vi "test.vi"() -> ()   [LabVIEW 2016]
panel:
  out "层数 2":string
  out "层数参数位置 2":i32
  out "总包数 2":i32
  out "当前包号 2":i32
  out "小时数据发送次数":i32
  out "大小":i32
  out "总包数":i32[](array[numeric])
  out "当前包号":i32[](array[numeric])
  out "行数":i32[](array[numeric])
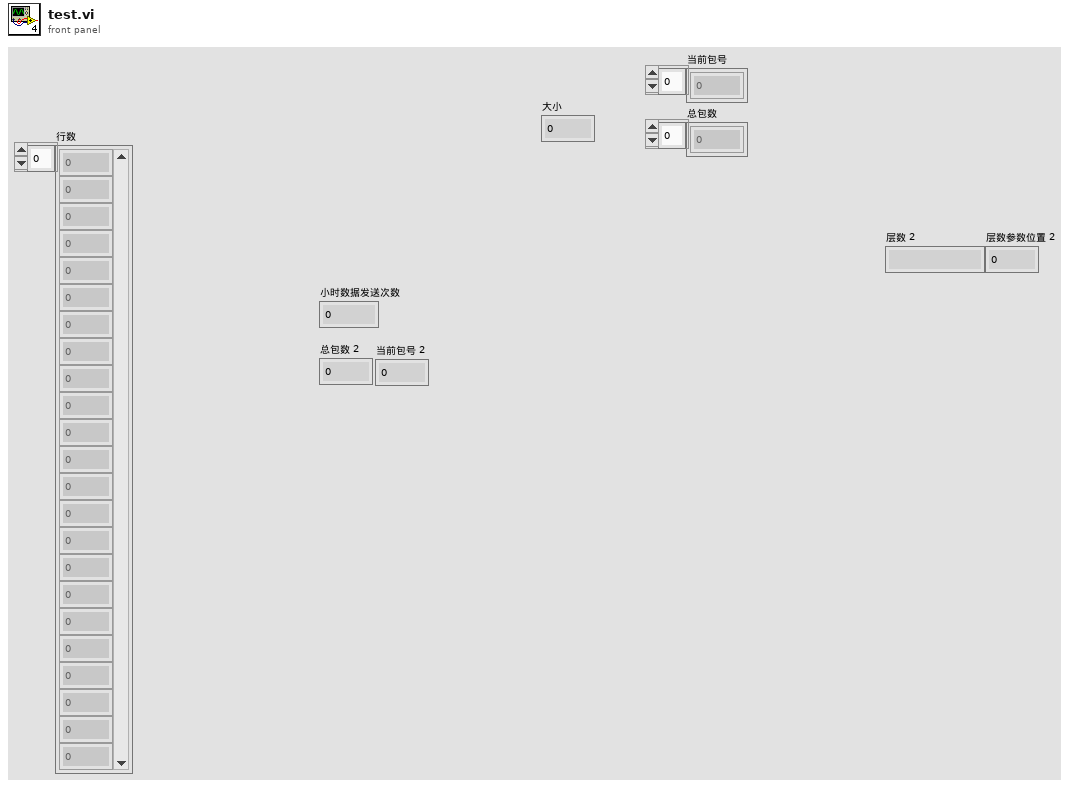
[diagram p1: front panel]
types:
  T1 = cluster{"CODMn":string, "CODCr":string, "DO":string, "铜":string, "PH":string, "氨氮":string, "比电导率":string, "水温":string, "COD":string, "浊度":string, "总氮":string, "总磷":string, "叶绿素a":string, "藻密度":string, "水位":string, "流速":string, "方向":string, "瞬时流量":string, "累积流量":string, "正累积流量":string, "负累积流量":string, "亚硝酸盐":string, "硫化物":string, "ORP":string, "铅":string, "镉":string, "锌":string, "镍":string, "锰":string, "汞":string, "气温":string, "气压":string, "风速":string, "风向":string, "空气温度":string, "相对湿度":string, "分钟雨量":string, "小时雨量":string, "日雨量":string, "累积雨量":string, "盐度":string, "磷酸盐":string, "硝氮":string, "氟化物":string, "挥发酚":string, "氯化物":string, "蓝绿藻":string, "余氯":string, "综合生物毒性":string, "艏向":string, "横摇":string, "纵摇":string, "分层标志":string, "层状态1":string, "层状态2":string, "水平平均流速":string, "流向":string, "北向流速分量":string, "东向流速分量":string, "垂直流速分量":string, "最大波高":string, "最大波周期":string, "1/10波高":string, "1/10波周期":string, "有效波高":string, "有效波周期":string, "平均波高":string, "平均波周期":string, "波向":string, "波个数":string, "水深":string}
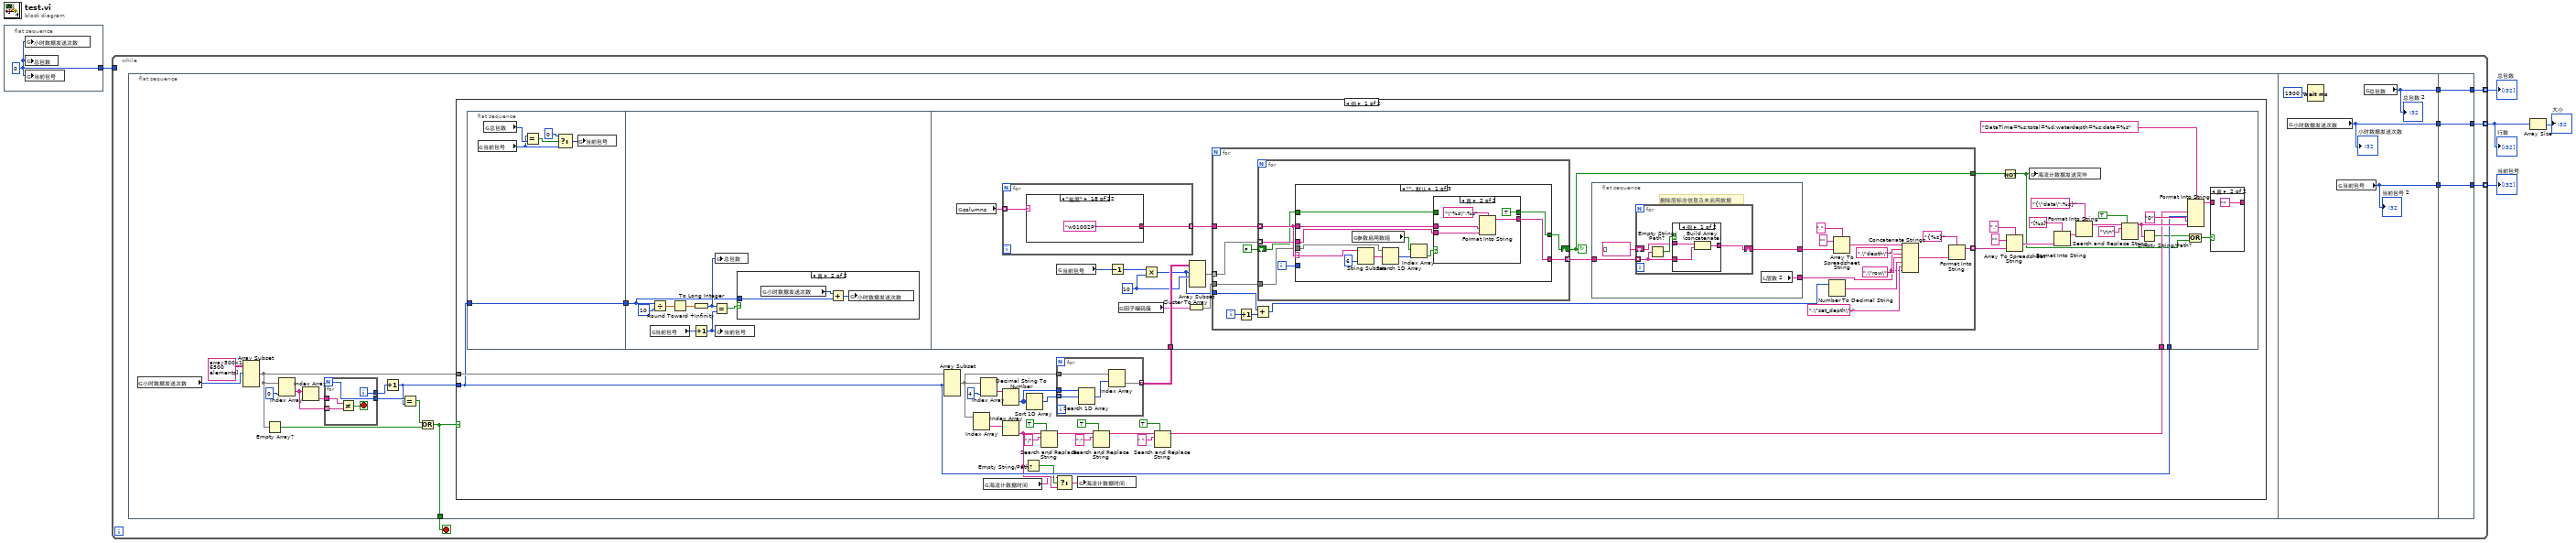
[diagram p0: block diagram]
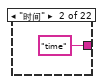
[diagram p5: hidden frame]
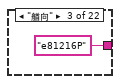
[diagram p6: hidden frame]
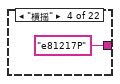
[diagram p7: hidden frame]
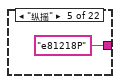
[diagram p8: hidden frame]
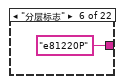
[diagram p9: hidden frame]
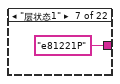
[diagram p10: hidden frame]
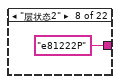
[diagram p11: hidden frame]
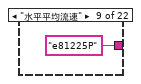
[diagram p12: hidden frame]
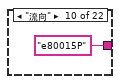
[diagram p13: hidden frame]
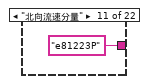
[diagram p14: hidden frame]
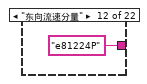
[diagram p15: hidden frame]
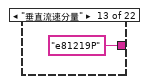
[diagram p16: hidden frame]
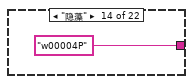
[diagram p17: hidden frame]
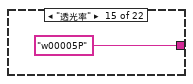
[diagram p18: hidden frame]
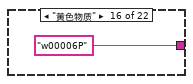
[diagram p19: hidden frame]
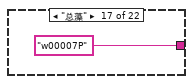
[diagram p20: hidden frame]
diagram:
  n1 = flat-sequence {
    tunnel: [w6] -> w1
    frame #0 {
      w6 = 0 ("小时数据发送次数")
      n2 = global write "全局 小时数据发送次数.vi" "小时数据发送次数"(w6) -> ()
      n3 = global write "全局 数据数组大小.vi" "总包数"(w6) -> ()
      n4 = global write "全局 数据数组大小.vi" "当前包号"(w6) -> ()
    }
  }
  n5 = while {
    tunnel: [w12] -> w3 mode=indexing
    tunnel: [w11] -> w5 mode=indexing
    tunnel: [w10] -> w4 mode=indexing
    tunnel: w1 -> [_]
    stop <- w13 stop-if-true
    n6 = flat-sequence {
      tunnel: [w14] -> w13
      tunnel: [w209] -> w9
      tunnel: [w208] -> w8
      tunnel: [w207] -> w7
      tunnel: [w210] -> w10
      tunnel: [w211] -> w11
      tunnel: [w212] -> w12
      tunnel: w9 -> [w212]
      tunnel: w8 -> [w211]
      tunnel: w7 -> [w210]
      frame #0 {
        n7 = global read "全局 小时数据发送次数.vi" "小时数据发送次数"() -> (w25:i32)
        n8 = Array Subset(array=string[][] array500x13[6500 elements] ("data"), index (row)=w25) -> (w15:string[][])  [unwired: 3 in]
        n9 = Empty Array?(array=w15) -> (empty?=w17:bool)
        n10 = Index Array(array=w15, index (col)=0 ("禁用的索引 (列)")) -> (element=w23:string[])  [unwired: 1 in]
        n11 = Index Array(array=w23) -> (element=w22:string)  [unwired: 1 in]
        n12 = for {
          N -> [w201]
          tunnel: w23 -> [w204] mode=indexing
          tunnel: w22 -> [w205]
          tunnel: [w202] -> w21
          tunnel: [w201] -> w20
          i -> [w202]
          stop <- w203 stop-if-true
          n13 = Not Equal?(x=w205, y=w204) -> (x != y?=w203:bool)
        }
        n14 = Increment(x=w21) -> (x+1=w19:i32)
        n15 = Equal?(x=w20, y=w19) -> (x = y?=w16:bool)
        n16 = Or(x=w16, y=w17) -> (x .or. y?=w14:bool)
        n17 = case shown="假" w14 {
          tunnel: w19 -> [w41 _]
          tunnel: w15 -> [w47 _]
          frame False {
            n18 = flat-sequence {
              tunnel: w41 -> [w54]
              tunnel: [w54] -> w48
              tunnel: w48 -> [w60]
              tunnel: w43 -> [w100]
              tunnel: w41 -> [w77]
              tunnel: w26 -> [w76]
              frame #0 {
                n19 = global read "全局 数据数组大小.vi" "当前包号"() -> (w57:i32)
                n20 = global read "全局 数据数组大小.vi" "总包数"() -> (w59:i32)
                n21 = Equal?(x=w57, y=w59) -> (x = y?=w58:bool)
                n22 = Select(t=0, s=w58, f=w57) -> (s? t:f=w55:i32)
                n23 = global write "全局 数据数组大小.vi" "当前包号"(w55) -> ()
              }
              frame #1 {
                n24 = global read "全局 数据数组大小.vi" "当前包号"() -> (w64:i32)
                n25 = Divide(x=w60, y=10) -> (x/y=w66:dbl)
                n26 = Round Toward +Infinity(x=w66) -> (ceil(x): smallest int >= x=w67:dbl)
                n27 = To Long Integer(number=w67) -> (32bit integer=w63:i32)
                n28 = Increment(x=w64) -> (x+1=w62:i32)
                n29 = Equal?(x=w63, y=w62) -> (x = y?=w61:bool)
                n30 = global write "全局 数据数组大小.vi" "总包数"(w63) -> ()
                n31 = global write "全局 数据数组大小.vi" "当前包号"(w62) -> ()
                n32 = case shown="真" w61 {
                  tunnel: w60 -> [_ w69]
                  frame False {
                  }
                  frame True {
                    n33 = global read "全局 小时数据发送次数.vi" "小时数据发送次数"() -> (w70:i32)
                    n34 = Add(x=w70, y=w69) -> (x+y=w68:i32)
                    n35 = global write "全局 小时数据发送次数.vi" "小时数据发送次数"(w68) -> ()
                  }
                }
              }
              frame #2 {
                w97 = 10 ("长度")
                n36 = global read "全局 所有参数.vi" "columns"() -> (w93:string[])
                n37 = for {
                  tunnel: w93 -> [w104] mode=indexing
                  tunnel: [w103] -> w92 mode=indexing
                  n38 = case shown="\"盐度\"" w104 {
                    tunnel: [_ "time" ("元素") "e81216P" "e81217P" "e81218P" "e81220P" "e81221P" "e81222P" "e81225P" "e80015P" "e81223P" "e81224P" "e81219P" "w00004P" "w00005P" "w00006P" "w00007P" "w01002P" "w01022P" "w81024P" "w81025P" "w81023P"] -> w103
                    frame "", Default {
                    }
                    frame "时间" {
                    }
                    frame "艏向" {
                    }
                    frame "横摇" {
                    }
                    frame "纵摇" {
                    }
                    frame "分层标志" {
                    }
                    frame "层状态1" {
                    }
                    frame "层状态2" {
                    }
                    frame "水平平均流速" {
                    }
                    frame "流向" {
                    }
                    frame "北向流速分量" {
                    }
                    frame "东向流速分量" {
                    }
                    frame "垂直流速分量" {
                    }
                    frame "隐藻" {
                    }
                    frame "透光率" {
                    }
                    frame "黄色物质" {
                    }
                    frame "总藻" {
                    }
                    frame "盐度" {
                    }
                    frame "蓝绿藻" {
                    }
                    frame "Fv/Fm" {
                    }
                    frame "PAR" {
                    }
                    frame "GPP" {
                    }
                  }
                }
                n39 = global read "全局 数据数组大小.vi" "当前包号"() -> (w99:i32)
                n40 = Decrement(x=w99) -> (x-1=w98:i32)
                n41 = global read "断电保存全局.vi" "因子编码簇"() -> (w96:T1)
                n42 = Multiply(x=w98, y=w97) -> (x*y=w91:i32)
                n43 = Cluster To Array(cluster=w96) -> (array=w95:string[])
                n44 = Array Subset(array=w100, index (row)=w91, length (row)=w97) -> (w94:string[][])  [unwired: 2 in]
                n45 = for {
                  tunnel: w94 -> [w146] mode=indexing
                  tunnel: w92 -> [w147]
                  tunnel: [w142] -> w78 mode=indexing
                  tunnel: w95 -> [w129]
                  tunnel: [w127] -> w75
                  tunnel: w91 -> [w126]
                  i -> [w141]
                  stop <- w127 continue-if-true
                  n46 = Increment(x=w141) -> (x+1=w133:i32)
                  n47 = Add(x=w126, y=w133) -> (x+y=w134:i32)
                  n48 = for {
                    tunnel: w147 -> [w165] mode=indexing
                    tunnel: w146 -> [w164] mode=indexing
                    tunnel: [w166] -> w132 mode=indexing
                    tunnel: w129 -> [w162]
                    shift-right: [w160] -> w127
                    shift-left: FALSE -> [w161]
                    i -> [w163]
                    n49 = case shown="\"\", 默认" w165 {
                      selector: w165 -> [w170 _ _]
                      tunnel: [w178 "" w199] -> w166
                      tunnel: w165 -> [w177 w190 w198]
                      tunnel: w164 -> [w176 w189 w194]
                      tunnel: w163 -> [_ w188 _]
                      tunnel: w162 -> [w175 _ _]
                      tunnel: w161 -> [w171 w186 w192]
                      tunnel: [w172 w186 w192] -> w160
                      frame "", Default {
                        n50 = global read "断电保存全局.vi" "参数启用数组"() -> (w174:bool[])
                        n51 = String Subset(string=w170, length (rest)=6 ("长度（剩余）")) -> (substring=w168:string)  [unwired: 1 in]
                        n52 = Search 1D Array(1D array=w175, element=w168) -> (index of element=w173:i32)  [unwired: 1 in]
                        n53 = Index Array(array=w174, index=w173) -> (element=w167:bool)
                        n54 = case shown="真" w167 {
                          tunnel: ["" w184] -> w178
                          tunnel: w177 -> [_ w183]
                          tunnel: w176 -> [_ w182]
                          tunnel: [w179 TRUE] -> w172
                          tunnel: w171 -> [w179 _]
                          frame False {
                          }
                          frame True {
                            n55 = Format Into String(format string="\"%s\":%s" ("格式字符串"), w183, w182) -> (resulting string=w184:string)  [unwired: 2 in, 1 out]
                          }
                        }
                      }
                      frame "e81220P" {
                        n56 = Format Into String(format string="\"%s\":%s" ("格式字符串"), w190, w189) -> ()  [unwired: 2 in, 2 out]
                        "层数 2" <- w189
                        "层数参数位置 2" <- w188
                      }
                      frame "time" {
                        n57 = Search and Replace String(replace all?=TRUE ("替换全部？(F)"), input string=w194, search string="/" ("搜索字符串"), replace string="-" ("替换字符串(\"\")")) -> (result string=w193:string)  [unwired: 4 in, 3 out]
                        n58 = Format Into String(format string="\"%s\":\"%s\"" ("格式字符串"), w198, w193) -> (resulting string=w199:string)  [unwired: 2 in, 1 out]
                      }
                    }
                  }
                  n59 = flat-sequence {
                    tunnel: w132 -> [w150]
                    tunnel: [w151] -> w131
                    tunnel: [w148] -> w130
                    frame #0 {
                      # "删除层标志信息及未启用数据"
                      n60 = for {
                        tunnel: w150 -> [w152] mode=indexing
                        shift-right: [w153] -> w148
                        shift-left: string[] [] -> [w154]
                        n61 = Empty String/Path?(string/path=w152) -> (empty?=w155:bool)
                        n62 = case shown="假" w155 {
                          tunnel: [w156 w159] -> w153
                          tunnel: w154 -> [w158 w159]
                          tunnel: w152 -> [w157 _]
                          frame False {
                            n63 = Build Array (concatenate)(w158, w157) -> (w156:string[])
                          }
                          frame True {
                          }
                        }
                      }
                      n64 = local read "层数 2"() -> (w151:string)
                    }
                  }
                  n65 = Number To Decimal String(number=w134) -> (decimal integer string=w138:string)  [unwired: 1 in]
                  n66 = Array To Spreadsheet String(delimiter (Tab)="," ("分隔符(Tab)"), array=w130, 3:"" ("格式字符串")) -> (spreadsheet string=w136:string)
                  n67 = Concatenate Strings(w136, ",\"depth\":", w131, ",\"row\":", w138, ",\"set_depth\":", w131) -> (w135:string)
                  n68 = Format Into String(format string="{%s}" ("格式字符串"), w135) -> (resulting string=w142:string)  [unwired: 2 in, 1 out]
                }
                n69 = Not(x=w75) -> (.not. x?=w73:bool)
                n70 = Array To Spreadsheet String(delimiter (Tab)="," ("分隔符(Tab)"), array=w78, 3:"" ("格式字符串")) -> (spreadsheet string=w85:string)
                n71 = global write "全局 数据数组大小.vi" "海流计数据发送完毕"(w73) -> ()
                n72 = Format Into String(format string="[%s]" ("格式字符串"), w85) -> (resulting string=w86:string)  [unwired: 2 in, 1 out]
                n73 = Format Into String(format string="{\"data\":%s}" ("格式字符串"), w86) -> (resulting string=w82:string)  [unwired: 2 in, 1 out]
                n74 = Search and Replace String(replace all?=TRUE ("替换全部？(F)"), input string=w82, search string="\r\n") -> (result string=w80:string)  [unwired: 5 in, 3 out]
                n75 = Empty String/Path?(string/path=w80) -> (empty?=w74:bool)
                n76 = Format Into String(format string="DataTime=%s;total=%d;waterdepth=%s;data=%s", w76, w77, "0" ("输入 3"), w80) -> (resulting string=w71:string)  [unwired: 2 in, 1 out]
                n77 = Compound Arithmetic op=OR ("复合运算")(w74, w73) -> (w72:bool)
                n78 = case shown="真" w72 {
                  tunnel: [w101 ""] -> _
                  tunnel: w71 -> [w101 _]
                  frame False {
                  }
                  frame True {
                  }
                }
              }
            }
            n79 = Array Subset(array=w47, length (row)=w41) -> (w27:string[][])  [unwired: 3 in]
            n80 = Index Array(array=w27) -> (element=w40:string[])  [unwired: 2 in]
            n81 = Index Array(array=w27, index (col)=4 ("禁用的索引 (列)")) -> (element=w46:string[])  [unwired: 1 in]
            n82 = global read "全局 水样时间.vi" "海流计数据时间"() -> (w29:string)
            n83 = Decimal String To Number(string=w46) -> (number=w45:i32[])  [unwired: 2 in, 1 out]
            n84 = Index Array(array=w40) -> (element=w30:string)  [unwired: 1 in]
            n85 = Empty String/Path?(string/path=w30) -> (empty?=w31:bool)
            n86 = Sort 1D Array(array=w45) -> (sorted array=w44:i32[])
            n87 = Search and Replace String(replace all?=TRUE ("替换全部？(F)"), input string=w30, search string="/" ("替换字符串(\"\")")) -> (result string=w35:string)  [unwired: 5 in, 3 out]
            n88 = Select(t=w29, s=w31, f=w30) -> (s? t:f=w28:string)
            n89 = for {
              tunnel: w45 -> [w53]
              tunnel: w44 -> [w52] mode=indexing
              tunnel: w27 -> [w51]
              tunnel: [w49] -> w43 mode=indexing
              n90 = Search 1D Array(1D array=w53, element=w52) -> (index of element=w50:i32)  [unwired: 1 in]
              n91 = Index Array(array=w51, index (row)=w50) -> (element=w49:string[])  [unwired: 1 in]
            }
            n92 = global write "全局 水样时间.vi" "海流计数据时间"(w28) -> ()
            n93 = Search and Replace String(replace all?=TRUE ("替换全部？(F)"), input string=w35, search string=":" ("替换字符串(\"\")")) -> (result string=w32:string)  [unwired: 5 in, 3 out]
            n94 = Search and Replace String(replace all?=TRUE ("替换全部？(F)"), input string=w32, search string=" " ("替换字符串(\"\")")) -> (result string=w26:string)  [unwired: 5 in, 3 out]
          }
          frame True {
          }
        }
      }
      frame #1 {
        n95 = global read "全局 小时数据发送次数.vi" "小时数据发送次数"() -> (w209:i32)
        "小时数据发送次数" <- w209
        n96 = Wait (ms)(milliseconds to wait=u32 1500 ("等待时间（毫秒）")) -> ()  [unwired: 1 out]
        n97 = global read "全局 数据数组大小.vi" "当前包号"() -> (w208:i32)
        "当前包号 2" <- w208
        n98 = global read "全局 数据数组大小.vi" "总包数"() -> (w207:i32)
        "总包数 2" <- w207
      }
      frame #2 {
      }
    }
  }
  "行数" <- w3
  "当前包号" <- w5
  "总包数" <- w4
  n99 = Array Size(array=w3) -> (size(s)=→"大小":i32)
